vi "Main_Individual.vi"(8 "error in":errorcluster caption="entrée d'erreur") -> (0 "error out":errorcluster caption="sortie d'erreur")   [LabVIEW 2026]
uses:
  APE codes/LabVIEW/LV13/Basic Example/cluster/tcp client action.ctl
panel:
  in  "Enable delay":bool
  in  "Get parameters":bool
  in  "Host":string="127.0.0.1"
  in  "Port":u16=51019
  in  "Disconnect":bool
  in  "Connect":bool
  in  "Delay (fs)":dbl
  in  "IR power (mW)":dbl
  in  "Signal power (mW)":dbl
  in  "Main shutter":bool
  in  "Signal shutter":bool
  in  "IR shutter":bool
  out "Sent string":string
  in  "Wavelength (nm)":dbl
  in  "Quit":bool
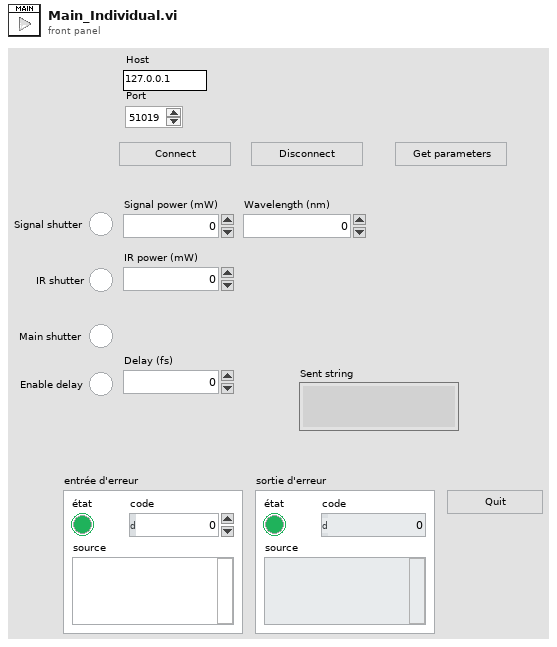
[diagram p1: front panel]
types:
  T1 = typedef "tcp client action.ctl" = enum16{"Connect", "Write", "Query", "Disconnect"}
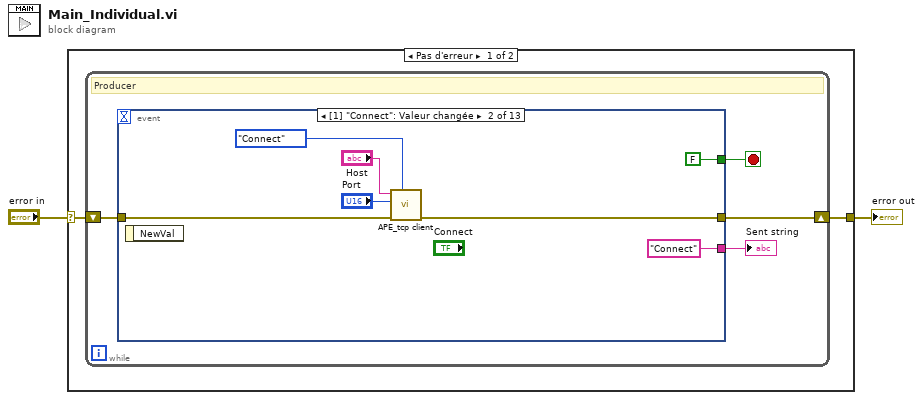
[diagram p0: block diagram]
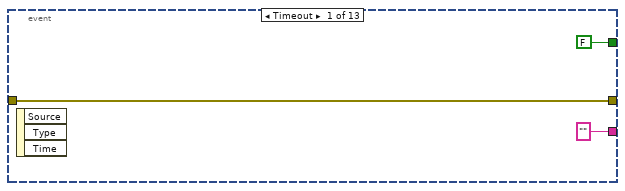
[diagram p2: hidden frame]
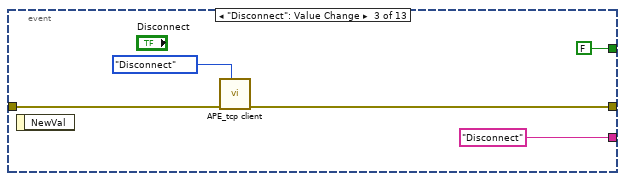
[diagram p3: hidden frame]
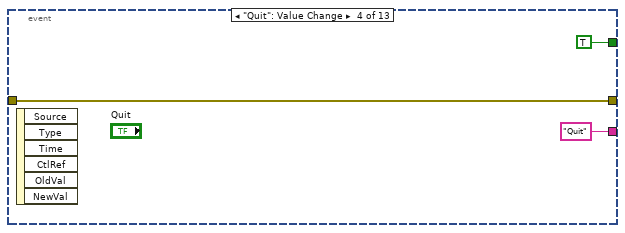
[diagram p4: hidden frame]
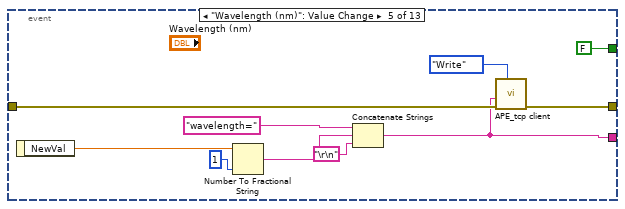
[diagram p5: hidden frame]
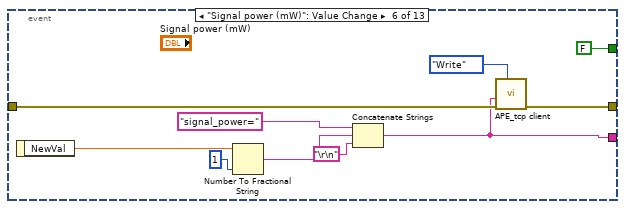
[diagram p6: hidden frame]
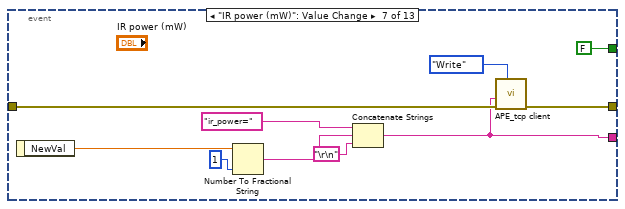
[diagram p7: hidden frame]
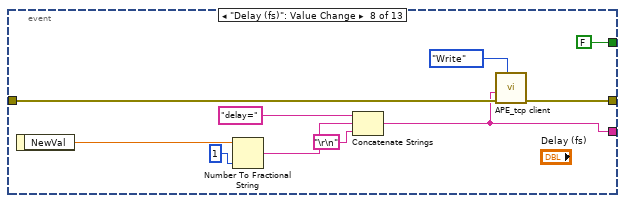
[diagram p8: hidden frame]
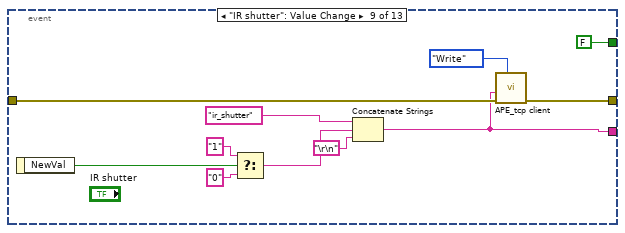
[diagram p9: hidden frame]
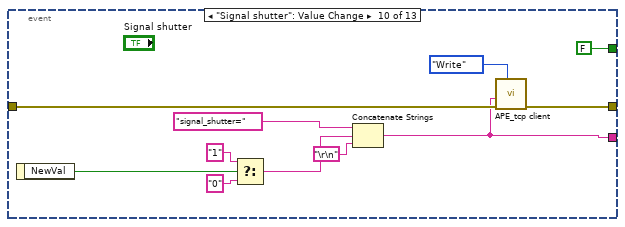
[diagram p10: hidden frame]
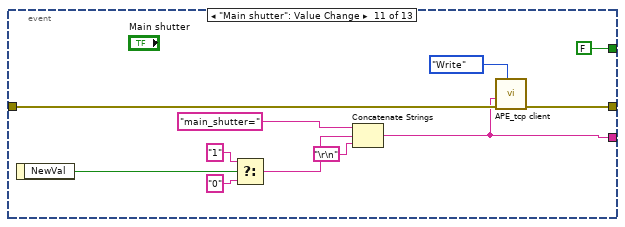
[diagram p11: hidden frame]
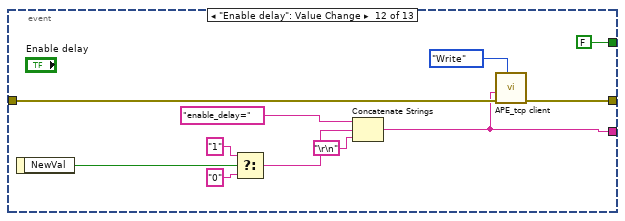
[diagram p12: hidden frame]
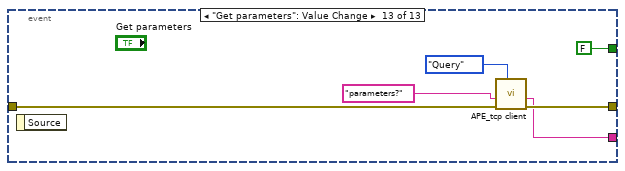
[diagram p13: hidden frame]
diagram:
  n1 = case shown="Pas d'erreur" "error in" {
    selector: "error in" -> [w4 w117]
    tunnel: [w3 w117] -> w1
    frame No Error {
      n2 = while {
        shift-right: [w7] -> w3
        shift-left: w4 -> [w8]
        stop <- w6 stop-if-true
        # "Producer"
        n3 = event shown="[1] \"Connect\": Valeur changée" {
          selector: _ -> [_ _ _ _ _ _ _ _ _ _ _ _ _]
          dyn-events: _ -> [_ _ _ _ _ _ _ _ _ _ _ _ _]
          timeout: _ -> [_ _ _ _ _ _ _ _ _ _ _ _ _]
          tunnel: w8 -> [w11 w15 w22 w26 w36 w46 w56 w66 w77 w88 w99 w110 w113]
          tunnel: [w11 w14 w21 w26 w35 w45 w55 w65 w76 w87 w98 w109 w115] -> w7
          tunnel: [FALSE FALSE FALSE TRUE FALSE FALSE FALSE FALSE FALSE FALSE FALSE FALSE FALSE] -> w6
          tunnel: ["" "Connect" "Disconnect" "Quit" w28 w38 w48 w58 w71 w82 w93 w104 w114] -> w5
          event Timeout {
            n4 = event-data() -> ()  [unwired: 1 in, 3 out]
          }
          event "Connect": Value Change {
            n5 = event-data() -> ()  [unwired: 1 in, 1 out]
            n6 = call "APE_tcp client.vi"("Action"=tcp_client_action."Connect", "error in"=w15, "TCP Port"="Port", "Host"="Host") -> ("error out"=w14:errorcluster)  [unwired: 6 in, 1 out]
          }
          event "Disconnect": Value Change {
            n7 = event-data() -> ()  [unwired: 1 in, 1 out]
            n8 = call "APE_tcp client.vi"("Action"=tcp_client_action."Disconnect", "error in"=w22) -> ("error out"=w21:errorcluster)  [unwired: 8 in, 1 out]
          }
          event "Quit": Value Change {
            n9 = event-data() -> ()  [unwired: 1 in, 6 out]
          }
          event "Wavelength (nm)": Value Change {
            n10 = event-data() -> ("NewVal"=w27:dbl)  [unwired: 1 in]
            n11 = Number To Fractional String(number=w27, precision (6)=i16 1 ("précision (6)")) -> (F-format string=w33:string)  [unwired: 2 in]
            n12 = Concatenate Strings("wavelength=" ("chaîne"), w33, "\r\n") -> (w28:string)
            n13 = call "APE_tcp client.vi"("Action"=tcp_client_action."Write", "error in"=w36, "Command"=w28) -> ("error out"=w35:errorcluster)  [unwired: 7 in, 1 out]
          }
          event "Signal power (mW)": Value Change {
            n14 = event-data() -> ("NewVal"=w37:dbl)  [unwired: 1 in]
            n15 = Number To Fractional String(number=w37, precision (6)=i16 1 ("précision (6)")) -> (F-format string=w43:string)  [unwired: 2 in]
            n16 = Concatenate Strings("signal_power=" ("chaîne"), w43, "\r\n") -> (w38:string)
            n17 = call "APE_tcp client.vi"("Action"=tcp_client_action."Write", "error in"=w46, "Command"=w38) -> ("error out"=w45:errorcluster)  [unwired: 7 in, 1 out]
          }
          event "IR power (mW)": Value Change {
            n18 = event-data() -> ("NewVal"=w47:dbl)  [unwired: 1 in]
            n19 = Number To Fractional String(number=w47, precision (6)=i16 1 ("précision (6)")) -> (F-format string=w53:string)  [unwired: 2 in]
            n20 = Concatenate Strings("ir_power=" ("chaîne"), w53, "\r\n") -> (w48:string)
            n21 = call "APE_tcp client.vi"("Action"=tcp_client_action."Write", "error in"=w56, "Command"=w48) -> ("error out"=w55:errorcluster)  [unwired: 7 in, 1 out]
          }
          event "Delay (fs)": Value Change {
            n22 = event-data() -> ("NewVal"=w57:dbl)  [unwired: 1 in]
            n23 = Number To Fractional String(number=w57, precision (6)=i16 1 ("précision (6)")) -> (F-format string=w63:string)  [unwired: 2 in]
            n24 = Concatenate Strings("delay=" ("chaîne"), w63, "\r\n") -> (w58:string)
            n25 = call "APE_tcp client.vi"("Action"=tcp_client_action."Write", "error in"=w66, "Command"=w58) -> ("error out"=w65:errorcluster)  [unwired: 7 in, 1 out]
          }
          event "IR shutter": Value Change {
            n26 = event-data() -> ("NewVal"=w70:bool)  [unwired: 1 in]
            n27 = Select(t="1", s=w70, f="0" ("cas faux")) -> (s? t:f=w67:string)
            n28 = Concatenate Strings("ir_shutter" ("chaîne"), w67, "\r\n") -> (w71:string)
            n29 = call "APE_tcp client.vi"("Action"=tcp_client_action."Write", "error in"=w77, "Command"=w71) -> ("error out"=w76:errorcluster)  [unwired: 7 in, 1 out]
          }
          event "Signal shutter": Value Change {
            n30 = event-data() -> ("NewVal"=w81:bool)  [unwired: 1 in]
            n31 = Select(t="1", s=w81, f="0" ("cas faux")) -> (s? t:f=w78:string)
            n32 = Concatenate Strings("signal_shutter=" ("chaîne"), w78, "\r\n") -> (w82:string)
            n33 = call "APE_tcp client.vi"("Action"=tcp_client_action."Write", "error in"=w88, "Command"=w82) -> ("error out"=w87:errorcluster)  [unwired: 7 in, 1 out]
          }
          event "Main shutter": Value Change {
            n34 = event-data() -> ("NewVal"=w92:bool)  [unwired: 1 in]
            n35 = Select(t="1", s=w92, f="0" ("cas faux")) -> (s? t:f=w89:string)
            n36 = Concatenate Strings("main_shutter=" ("chaîne"), w89, "\r\n") -> (w93:string)
            n37 = call "APE_tcp client.vi"("Action"=tcp_client_action."Write", "error in"=w99, "Command"=w93) -> ("error out"=w98:errorcluster)  [unwired: 7 in, 1 out]
          }
          event "Enable delay": Value Change {
            n38 = event-data() -> ("NewVal"=w103:bool)  [unwired: 1 in]
            n39 = Select(t="1", s=w103, f="0" ("cas faux")) -> (s? t:f=w100:string)
            n40 = Concatenate Strings("enable_delay=" ("chaîne"), w100, "\r\n") -> (w104:string)
            n41 = call "APE_tcp client.vi"("Action"=tcp_client_action."Write", "error in"=w110, "Command"=w104) -> ("error out"=w109:errorcluster)  [unwired: 7 in, 1 out]
          }
          event "Get parameters": Value Change {
            n42 = event-data() -> ()  [unwired: 1 in, 1 out]
            n43 = call "APE_tcp client.vi"("Action"=tcp_client_action."Query", "error in"=w113, "Command"="parameters?") -> ("error out"=w115:errorcluster, "Answer"=w114:string)  [unwired: 7 in]
          }
        }
        "Sent string" <- w5
      }
    }
    frame Error {
    }
  }
  "error out" <- w1
